vi "Initialize.vi"(8 "error in (no error)":errorcluster, 9 "Reset (True)":bool=TRUE, 10 "ID Query (True)":bool=TRUE, 11 "VISA resource name":refnum<visa-resource-name>) -> (0 "error out":errorcluster, 3 "VISA resource name out":refnum<visa-resource-name>)   [LabVIEW 2009, in "Tektronix AFG 3000 Series.lvlib"]
doc: "Establishes communication with the instrument and optionally performs an instrument identification query and/or an instrument reset. It also places the instrument in a default state needed for other instrument driver operations. Therefore, call this VI before calling other instrument driver VIs for this instrument. Generally, you need to call the <B>Initialize VI</B> only once at the beginning of an application."
uses:
  Tektronix AFG 3000 Series.lvlib
panel:
  # "(c) 2006-2009 National Instruments.  ALL RIGHTS RESERVED."
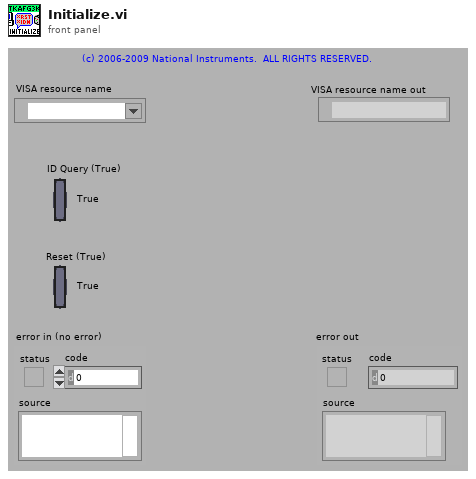
[diagram p1: front panel]
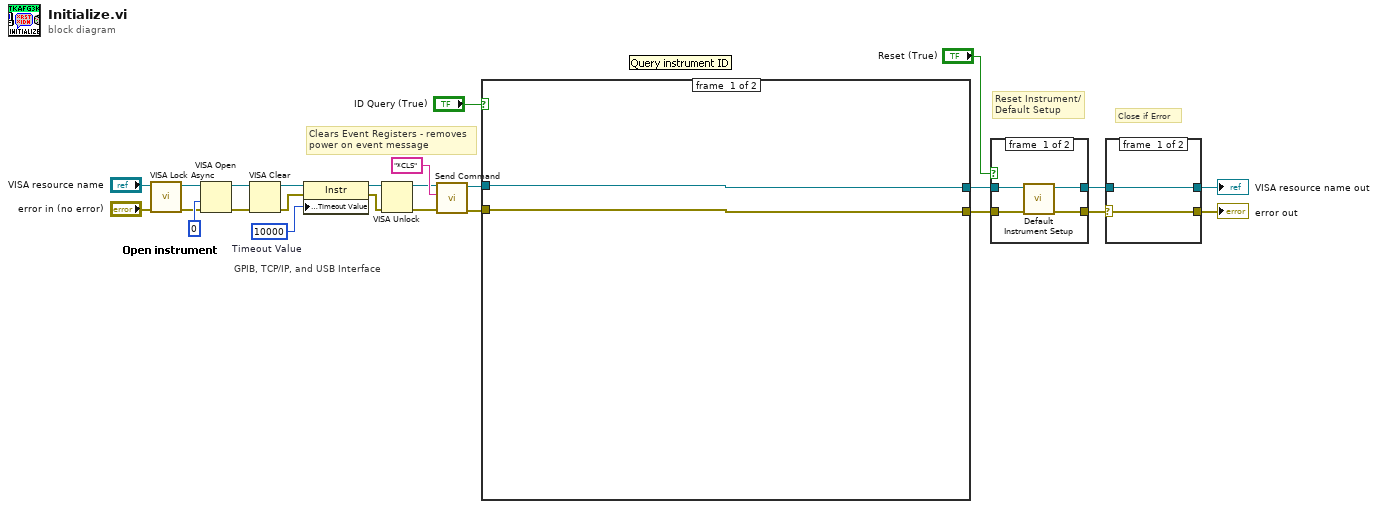
[diagram p0: block diagram]
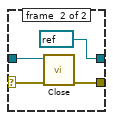
[diagram p2: hidden frame]
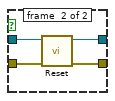
[diagram p3: hidden frame]
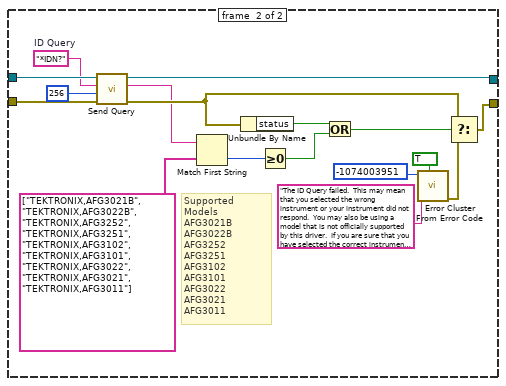
[diagram p4: hidden frame]
diagram:
  w16 = u32 10000  # Timeout Value
  # "Clears Event Registers - removes power on event message"
  # "GPIB, TCP/IP, and USB Interface"
  # "Close if Error"
  # "Reset Instrument/\nDefault Setup"
  n1 = call <vilib>:"VISA Lock Async.vi"("error in (no error)"="error in (no error)", "VISA resource name"="VISA resource name") -> ("error out"=w14:errorcluster, "VISA resource name out"=w13:refnum<visa-resource-name>)  [unwired: 1 in, 7 out]
  n2 = VISA Open(access mode=u32 0, error in (no error)=w14, VISA resource name=w13) -> (VISA resource name=w22:refnum<visa-resource-name>, error out=w21:errorcluster)  [unwired: 2 out]
  n3 = VISA Clear(VISA resource name=w22, error in (no error)=w21) -> (VISA resource name out=w6:refnum<visa-resource-name>, error out=w5:errorcluster)
  n4 = property class="Instr"(reference=w6, error in=w5, "General Settings:Timeout Value"=w16) -> (reference out=w4:refnum<visa-resource-name>, error out=w3:errorcluster)
  n5 = VISA Unlock(8:w3, 11:w4) -> (0:w1:errorcluster, 3:w2:refnum<visa-resource-name>)
  n6 = call "Send Command.vi"("error in (no error)"=w1, "write buffer"="*CLS", "VISA resource name"=w2) -> ("error out"=w7:errorcluster, "VISA resource name out"=w8:refnum<visa-resource-name>)  [unwired: 7 out]
  n7 = case shown="True" "ID Query (True)" {
    tunnel: [w26 w41] -> w9
    tunnel: [w27 w33] -> w10
    tunnel: w8 -> [w27 w34]
    tunnel: w7 -> [w26 w32]
    frame #0 {
    }
    frame #1 {
      w29 = "*IDN?"  # ID Query
      # "Supported Models\nAFG3021B\nAFG3022B\nAFG3252\nAFG3251\nAFG3102\nAFG3101\nAFG3022\nAFG3021\nAFG3011"
      n8 = call "Send Query.vi"("error in (no error)"=w32, "byte count (1024)"=u32 256, "write buffer"=w29, "VISA resource name"=w34) -> ("error out"=w31:errorcluster, "read buffer"=w30:string, "VISA resource name out"=w33:refnum<visa-resource-name>)  [unwired: 5 out]
      n9 = Match First String(2:string[] ["TEKTRONIX,AFG3021B", "TEKTRONIX,AFG3022B", "TEKTRONIX,AFG3252", "TEKTRONIX,AFG3251", "TEKTRONIX,AFG3102", "TEKTRONIX,AFG3101", "TEKTRONIX,AFG3022", "TEKTRONIX,AFG3021", "TEKTRONIX,AFG3011"] ("string array"), 3:w30) -> (0:w35:i32)  [unwired: 1 out]
      n10 = Unbundle By Name(w31) -> ("status"=w44:bool)
      n11 = Greater Or Equal To 0?(x=w35) -> (x >= 0?=w43:bool)
      n12 = Or(x=w44, y=w43) -> (x .or. y?=w42:bool)
      n13 = call <vilib>:"Error Cluster From Error Code.vi"("show call chain? (False)"=TRUE, "error message (\"\")"="The ID Query failed.  This may mean that you selected the wrong instrument or your instrument did not respond.  You may also be using a model that is not officially supported by this driver.  If you are sure that you have selected the correct instrument and it is responding, try disabling the ID Query." ("Source (VI Name)"), "error code (0)"=-1074003951 ("Code")) -> ("error out"=w36:errorcluster)  [unwired: 1 in, 5 out]
      n14 = Select(t=w31, s=w42, f=w36) -> (s? t:f=w41:errorcluster)
    }
  }
  n15 = case shown="False" "Reset (True)" {
    tunnel: [w47 w52] -> w17
    tunnel: w10 -> [w48 w50]
    tunnel: [w46 w51] -> w18
    tunnel: w9 -> [w45 w49]
    frame #0 {
      n16 = call "Default Instrument Setup.vi"("error in (no error)"=w45, "VISA resource name"=w48) -> ("error out"=w47:errorcluster, "VISA resource name out"=w46:refnum<visa-resource-name>)  [unwired: 8 out]
    }
    frame #1 {
      n17 = call "Reset.vi"("error in (no error)"=w49, "VISA resource name"=w50) -> ("error out"=w52:errorcluster, "VISA resource name out"=w51:refnum<visa-resource-name>)  [unwired: 8 out]
    }
  }
  n18 = case shown="Error" w17 {
    selector: w17 -> [w53 w56]
    tunnel: w18 -> [w54 w57]
    tunnel: [w54 refnum<visa-resource-name> refnum ("VISA resource name out")] -> w20
    tunnel: [w53 w58] -> w19
    frame #0 {
    }
    frame #1 {
      n19 = call "Close.vi"("error in (no error)"=w56, "VISA resource name"=w57) -> ("error out"=w58:errorcluster)  [unwired: 9 out]
    }
  }
  "VISA resource name out" <- w20
  "error out" <- w19
